vi "singleToneStore.vi"(6 "channel_name":string, 8 "error in (no error)":errorcluster, 9 "SingleTone.lvclass":refnum<class "SingleTone.lvclass">, 10 "action":enum16{"Write", "Read", "Reset"}(ring), 11 "SingleToneArray in":refnum<class "SingleToneArray.lvclass">) -> (0 "error out":errorcluster, 1 "SingleTone.lvclass out":refnum<class "SingleTone.lvclass">, 2 "found?":bool, 3 "SingleToneArray out":refnum<class "SingleToneArray.lvclass">)   [LabVIEW 2009, in "Tools.lvlib" / "Scripting.lvlib" / "SingleToneArray.lvclass"]
uses:
  SingleToneArray.lvclass
  SingleTone/SingleTone.lvclass
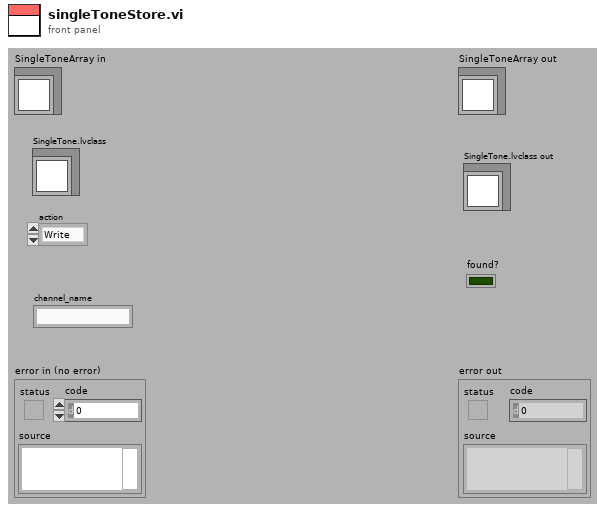
[diagram p1: front panel]
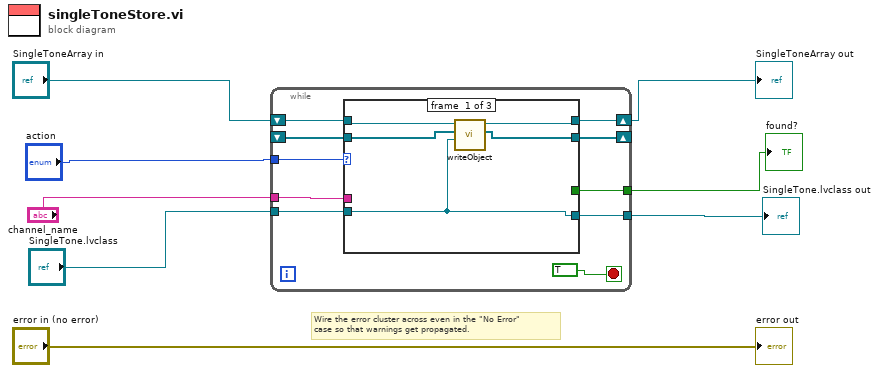
[diagram p0: block diagram]
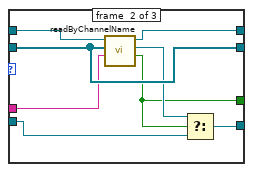
[diagram p2: hidden frame]
diagram:
  # "Wire the error cluster across even in the \"No Error\"\ncase so that warnings get propagated."
  n1 = while {
    tunnel: "action" -> [w17]
    shift-right: [w14] -> _
    shift-left: _ -> [w16]
    tunnel: "SingleTone.lvclass" -> [w15]
    shift-right: [w12] -> w4
    shift-left: "SingleToneArray in" -> [w13]
    tunnel: [w11] -> w2
    tunnel: "channel_name" -> [w10]
    tunnel: [w9] -> w1
    stop <- TRUE stop-if-true
    n2 = case shown="\"Reset\"" w17 {
      tunnel: w16 -> [w21 w29 _]
      tunnel: w15 -> [w19 w26 _]
      tunnel: [w20 w29 _] -> w14
      tunnel: w13 -> [w23 w31 w32]
      tunnel: [w22 w30 w32] -> w12
      tunnel: [w19 w25 _] -> w11
      tunnel: w10 -> [_ w28 _]
      tunnel: [_ w24 _] -> w9
      frame #0 {
        n3 = call "writeObject.vi"("SingleTone.lvclass"=w19, "Array"=w21, "SingleToneArray in"=w23) -> ("Array out"=w20:refnum<class "SingleTone.lvclass">[], "SingleToneArray out"=w22:refnum<class "SingleToneArray.lvclass">)  [unwired: 6 in, 1 out]
      }
      frame #1 {
        n4 = call "readByChannelName.vi"("channel_name"=w28, "Array"=w29, "SingleToneArray in"=w31) -> ("found?"=w24:bool, "SingleTone.lvclass"=w27:refnum<class "SingleTone.lvclass">, "SingleToneArray out"=w30:refnum<class "SingleToneArray.lvclass">)  [unwired: 5 in, 1 out]
        n5 = Select(t=w27, s=w24, f=w26) -> (s? t:f=w25:refnum<class "SingleTone.lvclass">)
      }
      frame #2 {
      }
    }
  }
  "SingleToneArray out" <- w4
  "SingleTone.lvclass out" <- w2
  "found?" <- w1
  "error out" <- "error in (no error)"
